vi "Delete Queue (wait).vi"(0 "queue":refnum<queue>, 11 "error in (no error)":errorcluster) -> (15 "error out":errorcluster)   [LabVIEW 2020]
panel:
  in  "timeout(ms)":u32=1000
  in  "poll interval(ms)":u32=10
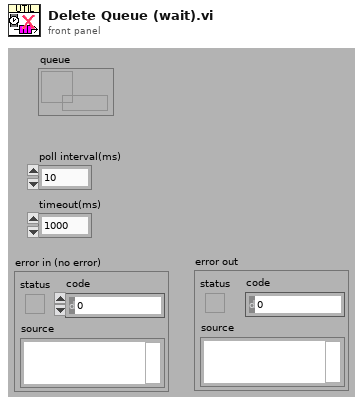
[diagram p1: front panel]
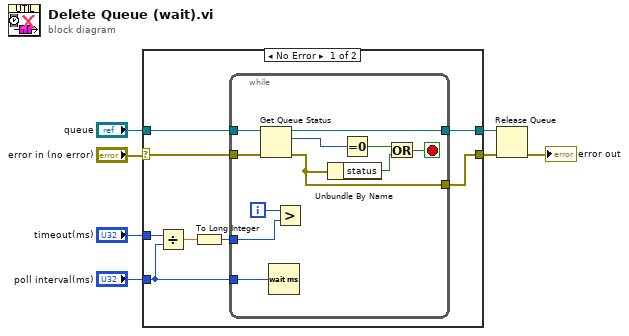
[diagram p0: block diagram]
diagram:
  n1 = case shown="No Error" "error in (no error)" {
    selector: "error in (no error)" -> [w10 w28]
    tunnel: "queue" -> [w15 w27]
    tunnel: "timeout(ms)" -> [w14 _]
    tunnel: "poll interval(ms)" -> [w13 _]
    tunnel: [w9 w28] -> w2
    tunnel: [w8 w27] -> w3
    frame No Error {
      n2 = Divide(x=w14, y=w13) -> (x/y=w12:dbl)
      n3 = To Long Integer(number=w12) -> (32bit integer=w11:i32)
      n4 = while {
        tunnel: w15 -> [w26]
        tunnel: w10 -> [w25]
        tunnel: [w20] -> w9
        tunnel: w13 -> [w19]
        tunnel: w11 -> [w17]
        tunnel: [w16] -> w8
        i -> [w18]
        stop <- w22 stop-if-true
        n5 = Get Queue Status(queue=w26, error in (no error)=w25) -> (queue out=w16:refnum<queue>, # pending remove=w24:i32, error out=w20:errorcluster)  [unwired: 1 in, 5 out]
        n6 = Wait (ms)(milliseconds to wait=w19) -> ()  [unwired: 1 out]
        n7 = Greater?(x=w18, y=w17) -> ()  [unwired: 1 out]
        n8 = Unbundle By Name(w20) -> ("status"=w21:bool)
        n9 = Equal To 0?(x=w24) -> (x = 0?=w23:bool)
        n10 = Or(x=w23, y=w21) -> (x .or. y?=w22:bool)
      }
    }
    frame Error {
    }
  }
  n11 = Release Queue(queue=w3, error in (no error)=w2) -> (error out=→"error out":errorcluster)  [unwired: 1 in, 2 out]
